vi "HighLvCtrl_Loop.vi"(7 "Processor (-2:auto)":i32=-2, 8 "error in (no error)":errorcluster, 11 "Cluster":T4) -> (0 "error out":errorcluster)   [LabVIEW 2015]
uses:
  Classes/CAlex2/CAlex2.lvclass
  Classes/ForceField/ForceField.lvclass
  <vilib>/Analysis/Matrix/Datatypes/RealMatrix.ctl
  <vilib>/Platform/TimedLoop/XDataNode/timing_clust.ctl
  <vilib>/Platform/TimedLoop/XDataNode/nitl_modes.ctl
  <vilib>/Platform/TimedLoop/XDataNode/wakeup.ctl
  Classes/CAlex2/TypeDef/LowerBodyDim.ctl
  Classes/ForceField/TypeDef/FF_Gains.ctl
  Classes/MotorControl/TypeDef/MotorMode.ctl
  Classes/ForceField/FF_SetGains.vi
  <vilib>/Platform/TimedLoop/XDataNode/XDataNode.xnode
  <vilib>/Platform/TimedLoop/XDataNode/XDNodeRunTimeDep.lvlib
  Classes/SerialChain-Cable/SerialChain-Cable.lvclass
  <vilib>/Analysis/NI_AALBase.lvlib
  <vilib>/Analysis/Matrix/NI_Matrix.lvlib
  <vilib>/GoldZinc Software/auzn custom VIs/CustomVI.lvlib
  <vilib>/Analysis/baseanly.llb/A x Vector.vi
panel:
  in  "history length (100)":i32=50
  in  "Thigh Reference (to Hip)":enum16{"Hip", "Ground"}(ring)=enum."Ground"
  in  "LP":bool
  out "QPSolved":bool
  out "Torque Error":dbl[](array[numeric]) format="%#.4f"
  in  "dt":dbl=0.01 format="%#_13g"
  out "Torque":T1(graph)
  out "Joint Angles (deg)":T2(graph)
  out "Desired Torque":dbl[](array[numeric]) format="%#.4f"
  out "Actual Torque":dbl[](array[numeric]) format="%#.4f"
  in  "LockedJoints":i32[](array[numeric])=[2, 1]
  out "Jacobian for Cables":T3 format="%#.3f"
  in  "TargetF(N)":dbl=15.0 format="%#_13g"
  in  "LP fc":dbl=10.0 format="%0.3f"
  in  "QPmode":enum16{"tight", "loose", "adv"}(ring)=enum."adv"
  in  "F range":cluster{"Fmin":dbl, "Fmax":dbl}[](array[cluster])=[{"Fmin"=15.0, "Fmax"=80.0}, {"Fmin"=10.0, "Fmax"=80.0}, {"Fmin"=10.0, "Fmax"=80.0}, {"Fmin"=10.0, "Fmax"=80.0}]
  # "In Cable Order, Not Motor Order"
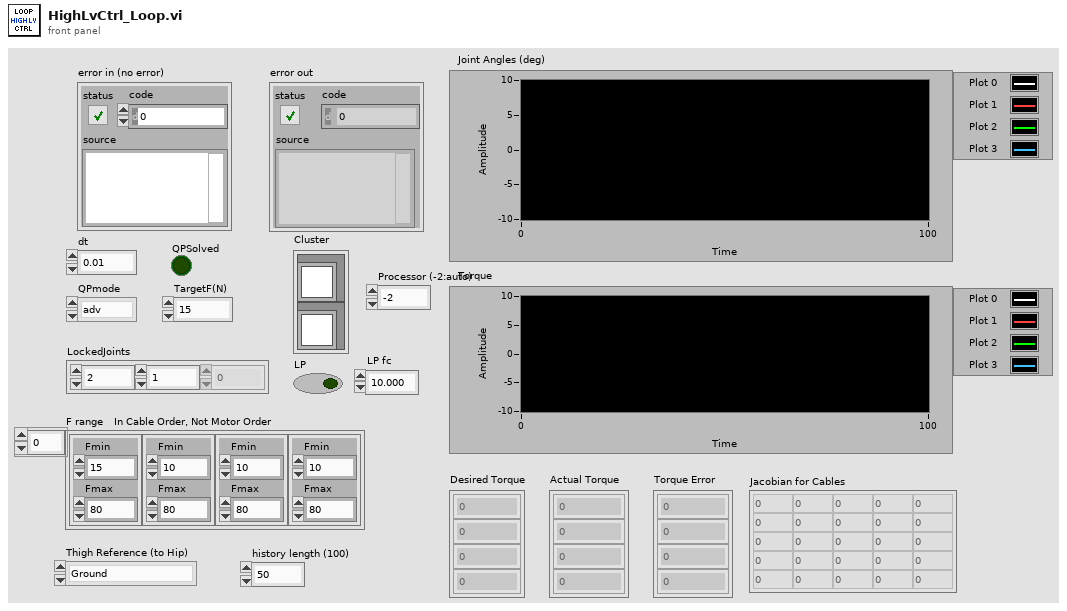
[diagram p1: front panel]
types:
  T1 = cluster{"[0]":dbl, "[1]":dbl, "[2]":dbl, "[3]":dbl, "[4]":dbl, "[5]":dbl, "[6]":dbl, "[7]":dbl, "[8]":dbl}
  T2 = cluster{"Joint Angles (rad)[0]":dbl, "Joint Angles (rad)[1]":dbl, "Joint Angles (rad)[2]":dbl, "Joint Angles (rad)[3]":dbl}
  T3 = typedef "NI_Matrix.lvlib/RealMatrix.ctl" = dbl[][]
  T4 = cluster{"CAlex":refnum<class "CAlex2.lvclass">, "ForceField":refnum<class "ForceField.lvclass">}
  T5 = typedef "XDNodeRunTimeDep.lvlib/timing_clust.ctl" = cluster{"Expected End [f-1]":u64, "Actual End [f-1]":u64, "Finished Late? [f-1]":bool, "Expected End [i-1]":u64, "Actual End [i-1]":u64, "Finished Late? [i-1]":bool, "Expected Start [i]":u64, "Actual Start [i]":u64, "Expected Start [f]":u64, "Actual Start [f]":u64, "Source Name":string, "Structure Name":string, "Period":i64, "Deadline":i64, "Offset":i64, "Start":i64, "Priority":i32, "Timeout":i32, "Mode":T6, "Wakeup Reason":T7, "Error":errorcluster, "Source Type":string, "Secondary Source Type":string, "Global End Time":u64, "Global Start Time":u64, "Frame Duration":u64, "Iteration Duration":u64, "Assigned CPU":i32, "I/O Scan Engine Mode":u32}
  T6 = typedef "XDNodeRunTimeDep.lvlib/nitl_modes.ctl" = enum32{"No Change", "Process missed periods, maintain original phase", "Discard missed periods, maintain original phase", "Process missed periods, ignore original phase", "Discard missed periods, ignore original phase"}
  T7 = typedef "XDNodeRunTimeDep.lvlib/wakeup.ctl" = enum32{"Normal", "Aborted", "Asynchronous wakeup", "Timing source error", "Timed loop error", "Timeout"}
  T8 = typedef "ForceField.lvclass/FF_Gains.ctl" = cluster{"Kn":dbl, "Dn":dbl, "Kt":dbl, "Dt":dbl, "Kd":dbl, "Ns":dbl}
  T9 = typedef "CAlex2.lvclass/LowerBodyDim.ctl" = cluster{"BodyDim":cluster{"ThighLt (m)":dbl, "ShankLt (m)":dbl, "HipWd (m)":dbl}, "BodyWt":cluster{"Thigh (kg)":dbl, "Shank (kg)":dbl}, "Cuff Loc":cluster{"HipCuffWd (m)":dbl, "HipCuffHt (m)":dbl, "HipFwdShift (m)":dbl, "ThighToKnee (m)":dbl, "ThighCuffDist (m)":dbl, "ShankToKnee (m)":dbl}}
  T10 = typedef "SerialChain.lvclass/PointOnBody.ctl" = cluster{"Coord4":dbl[], "ID":i32}
  T11 = cluster{"EndEffPos":T10, "Array of Double":dbl[]}
  T12 = typedef "MotorControl.lvclass/MotorMode.ctl" = enum16{"Idle", "FF", "PID"}
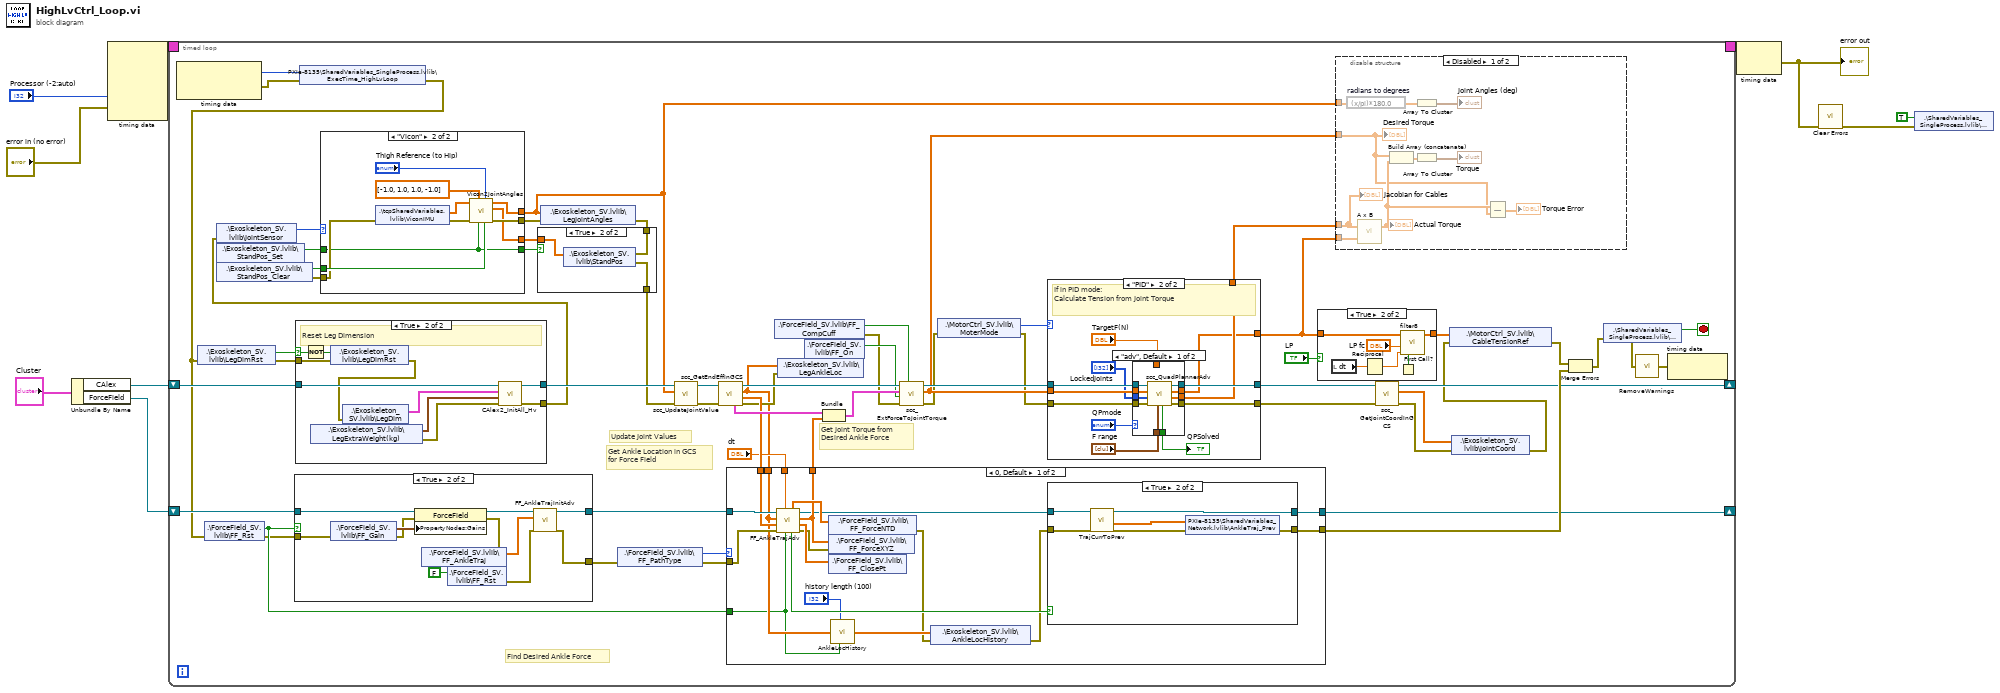
[diagram p0: block diagram]
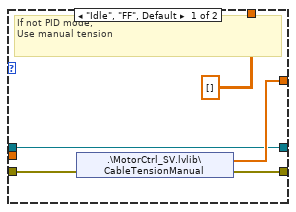
[diagram p4: hidden frame]
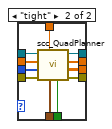
[diagram p5: hidden frame]
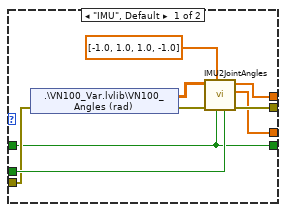
[diagram p6: hidden frame]
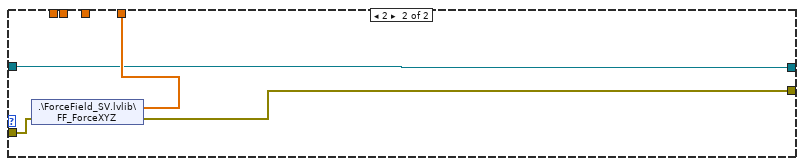
[diagram p11: hidden frame]
diagram:
  n1 = Unbundle By Name("Cluster") -> ("CAlex"=w6:refnum<class "CAlex2.lvclass">, "ForceField"=w5:refnum<class "ForceField.lvclass">)
  n2 = node-c288("Processor (-2:auto)", "error in (no error)") -> (w10:T5)  [unwired: 3 in]
  n3 = timed-loop {
    timing: w10 -> [_]
    timing-out: [_] -> w9
    shift-right: [w15] -> _
    shift-left: w6 -> [w74]
    shift-right: [w36] -> _
    shift-left: w5 -> [w71]
    stop <- w38 stop-if-true
    # "Get Joint Torque from Desired Ankle Force"
    # "Find Desired Ankle Force"
    # "Get Ankle Location in GCS for Force Field"
    # "Update Joint Values"
    n4 = node-c288() -> (w73:i64, w72:errorcluster)  [unwired: 1 in]
    n5 = shared-variable "PXIe-8135\\SharedVariables_SingleProcess.lvlib\\ExecTime_HighLvLoop"(w73, error in=w72) -> (error out=w33:errorcluster)
    n6 = shared-variable ".\\Exoskeleton_SV.lvlib\\LegDimRst"(error in=w33) -> (w52:bool, error out=w66:errorcluster)
    n7 = shared-variable ".\\ForceField_SV.lvlib\\FF_Rst"(error in=w33) -> (w49:bool, error out=w48:errorcluster)
    n8 = case shown="True" w49 {
      tunnel: w71 -> [w154 w166]
      tunnel: [w154 w165] -> w65
      tunnel: w48 -> [w153 w161]
      tunnel: [w153 w155] -> w51
      frame False {
      }
      frame True {
        n9 = shared-variable ".\\ForceField_SV.lvlib\\FF_Gain"(error in=w161) -> (w164:T8, error out=w159:errorcluster)
        n10 = property class="ForceField"(reference=w166, error in=w159, "PropertyNodes:Gains"=w164) -> (reference out=w163:refnum<class "ForceField.lvclass">, error out=w158:errorcluster)
        n11 = shared-variable ".\\ForceField_SV.lvlib\\FF_AnkleTraj"(error in=w158) -> (w162:dbl[][], error out=w157:errorcluster)
        n12 = shared-variable ".\\ForceField_SV.lvlib\\FF_Rst"(FALSE ("FFRst"), error in=w157) -> (error out=w156:errorcluster)
        n13 = call "FF_AnkleTrajInitAdv.vi"("error in (no error)"=w156, "AnkleTraj"=w162, "Force Field Controller in"=w163) -> ("error out"=w155:errorcluster, "Force Field Controller out"=w165:refnum<class "ForceField.lvclass">)  [unwired: 6 in, 1 out]
      }
    }
    n14 = case shown="True" w52 {
      selector: w52 -> [_ w174]
      tunnel: w74 -> [w168 w179]
      tunnel: [w168 w178] -> w67
      tunnel: w66 -> [w167 w177]
      tunnel: [w167 w172] -> w28
      frame False {
      }
      frame True {
        # "Reset Leg Dimension"
        n15 = Not(x=w174) -> (.not. x?=w175:bool)
        n16 = shared-variable ".\\Exoskeleton_SV.lvlib\\LegDimRst"(w175, error in=w177) -> (error out=w171:errorcluster)
        n17 = shared-variable ".\\Exoskeleton_SV.lvlib\\LegDim"(error in=w171) -> (w176:T9, error out=w170:errorcluster)
        n18 = shared-variable ".\\Exoskeleton_SV.lvlib\\LegExtraWeight(kg)"(error in=w170) -> (w173:cluster{"Thigh":dbl, "Shank":dbl}, error out=w169:errorcluster)
        n19 = call-dynamic "CAlex2_InitAll_Hv.vi"("error in (no error)"=w169, "ExtraWeight(kg)"=w173, "LegProperties"=w176, "CAlex2 in"=w179) -> ("error out"=w172:errorcluster, "CAlex2 out"=w178:refnum<class "CAlex2.lvclass">)  [unwired: 6 in]
      }
    }
    n20 = shared-variable ".\\Exoskeleton_SV.lvlib\\JointSensor"(error in=w28) -> (w42:enum16{"IMU", "Vicon"}, error out=w34:errorcluster)
    n21 = shared-variable ".\\Exoskeleton_SV.lvlib\\StandPos_Set"(error in=w34) -> (w53:bool, error out=w40:errorcluster)
    n22 = shared-variable ".\\Exoskeleton_SV.lvlib\\StandPos_Clear"(error in=w40) -> (w54:bool, error out=w41:errorcluster)
    n23 = case shown="\"Vicon\"" w42 {
      tunnel: w54 -> [w129 w141]
      tunnel: w53 -> [w124 w134]
      tunnel: [w128 w139] -> w46
      tunnel: [w127 w142] -> w45
      tunnel: w41 -> [w126 w138]
      tunnel: [w125 w135] -> w24
      tunnel: [w124 w134] -> w23
      frame "IMU", Default {
        n24 = shared-variable ".\\VN100_Var.lvlib\\VN100_Angles (rad)"(error in=w126) -> (w130:dbl[][], error out=w131:errorcluster)
        n25 = call "IMU2JointAngles.vi"("ResetZeroOrient"=w129, "SetZeroOrient"=w124, "JointAngleDir"=dbl[] [-1.0, 1.0, 1.0, -1.0], "error in (no error)"=w131, "IMU in (rad)"=w130) -> ("error out"=w127:errorcluster, "StandPos"=w125:dbl[], "Joint Angles (rad)"=w128:dbl[])  [unwired: 4 in]
      }
      frame "Vicon" {
        n26 = shared-variable ".\\tcpSharedVariables.lvlib\\ViconIMU"(error in=w138) -> (w137:dbl[], error out=w136:errorcluster)
        n27 = call "Vicon2JointAngles.vi"("Reset"=w141, "Thigh Reference (to Hip)"="Thigh Reference (to Hip)", "SetZeroOrient"=w134, "JointAngleDir([-1,1,1,-1])"=dbl[] [-1.0, 1.0, 1.0, -1.0], "error in (no error)"=w136, "ViconIMU in (rad)"=w137) -> ("error out"=w142:errorcluster, "StandPos"=w135:dbl[], "Joint Angles (rad)"=w139:dbl[])  [unwired: 3 in]
      }
    }
    n28 = shared-variable ".\\Exoskeleton_SV.lvlib\\LegJointAngles"(w46, error in=w45) -> (error out=w26:errorcluster)
    n29 = case shown="True" w23 {
      tunnel: w26 -> [w82 w85]
      tunnel: [w82 w84] -> w25
      tunnel: w24 -> [_ w83]
      frame False {
      }
      frame True {
        n30 = shared-variable ".\\Exoskeleton_SV.lvlib\\StandPos"(w83, error in=w85) -> (error out=w84:errorcluster)
      }
    }
    n31 = shared-variable ".\\ForceField_SV.lvlib\\FF_PathType"(error in=w51) -> (w61:i8, error out=w60:errorcluster)
    n32 = call-dynamic "scc_UpdateJointValue.vi"("error in (no error)"=w25, "JointValue (rad|m)"=w46, "C-Alex in"=w67) -> ("error out"=w18:errorcluster, "C-Alex out"=w19:refnum<class "CAlex2.lvclass">)  [unwired: 7 in]
    n33 = call "scc_GetEndEffInGCS.vi"("error in (no error)"=w18, "SerialChain_Cable in"=w19) -> ("error out"=w50:errorcluster, "Vendeff(GCS)"=w62:dbl[], "Pendeff(GCS)"=w11:dbl[], "SerialChain_Cable out"=w69:refnum<class "CAlex2.lvclass">, "EndEffPos"=w70:T10)  [unwired: 5 in]
    n34 = case shown="0, Default" w61 {
      tunnel: w65 -> [w199 w210]
      tunnel: w60 -> [w195 w209]
      tunnel: [w188 w210] -> w36
      tunnel: [w194 w211] -> w63
      tunnel: w11 -> [w184 _]
      tunnel: w62 -> [w191 _]
      tunnel: "dt" -> [w190 _]
      tunnel: w49 -> [w183 _]
      tunnel: [w187 w208] -> w37
      frame 0, Default {
        n35 = call "FF_AnkleTrajAdv.vi"("Init"=w183, "dt"=w190, "error in (no error)"=w195, "AnkleVelocity"=w191, "AnkleInGCS"=w184, "Force Field Controller in"=w199) -> ("error out"=w193:errorcluster, "ClosestPoint"=w197:dbl[], "ForceXYZ"=w194:dbl[], "Force Field Controller out"=w189:refnum<class "ForceField.lvclass">, "UpdateTrajPrev"=w186:bool, "ForceNTD"=w198:dbl[])
        n36 = shared-variable ".\\ForceField_SV.lvlib\\FF_ForceXYZ"(w194, error in=w193) -> (error out=w192:errorcluster)
        n37 = shared-variable ".\\ForceField_SV.lvlib\\FF_ClosePt"(w197, error in=w192) -> (error out=w196:errorcluster)
        n38 = shared-variable ".\\ForceField_SV.lvlib\\FF_ForceNTD"(w198, error in=w196) -> (error out=w182:errorcluster)
        n39 = call "AnkleLocHistory.vi"("history length (100)"="history length (100)", "AnkleLoc"=w184, "initialize"=w183) -> ("AnkleLoc"=w185:dbl[][])  [unwired: 2 in]
        n40 = shared-variable ".\\Exoskeleton_SV.lvlib\\AnkleLocHistory"(w185, error in=w182) -> (error out=w181:errorcluster)
        n41 = case shown="True" w186 {
          tunnel: w189 -> [w201 w206]
          tunnel: [w201 w207] -> w188
          tunnel: w181 -> [w200 w204]
          tunnel: [w200 w202] -> w187
          frame False {
          }
          frame True {
            n42 = call "TrajCurrToPrev.vi"("error in (no error)"=w204, "ForceField"=w206) -> ("error out"=w203:errorcluster, "AnkleTraj_array"=w205:dbl[][], "ForceField 2"=w207:refnum<class "ForceField.lvclass">)  [unwired: 6 in, 1 out]
            n43 = shared-variable "PXIe-8135\\SharedVariables_Network.lvlib\\AnkleTraj_Prev"(w205, error in=w203) -> (error out=w202:errorcluster)
          }
        }
      }
      frame 2 {
        n44 = shared-variable ".\\ForceField_SV.lvlib\\FF_ForceXYZ"(error in=w209) -> (w211:dbl[], error out=w208:errorcluster)
      }
    }
    n45 = shared-variable ".\\Exoskeleton_SV.lvlib\\LegAnkleLoc"(w11, error in=w50) -> (error out=w58:errorcluster)
    n46 = shared-variable ".\\ForceField_SV.lvlib\\FF_On"(error in=w58) -> (w57:bool, error out=w59:errorcluster)
    n47 = shared-variable ".\\ForceField_SV.lvlib\\FF_CompCuff"(error in=w59) -> (w35:bool, error out=w56:errorcluster)
    n48 = Bundle("EndEffPos"=w70, "Array of Double"=w63) -> (w64:T11)  [unwired: 1 in]
    n49 = call "scc_ExtForceToJointTorque.vi"("CuffWtComp?(F)"=w35, "error in (no error)"=w56, "ExternalForce(T)"=w57, "External Force (In GCS)"=w64, "SerialChain_Cable in"=w69) -> ("error out"=w29:errorcluster, "DesiredTorque(Nm)"=w44:dbl[], "SerialChain_Cable out"=w68:refnum<class "CAlex2.lvclass">)  [unwired: 4 in]
    n50 = shared-variable ".\\MotorCtrl_SV.lvlib\\MoterMode"(error in=w29) -> (w31:T12, error out=w30:errorcluster)
    n51 = case shown="\"PID\"" w31 {
      tunnel: [w89 w102] -> w17
      tunnel: w30 -> [w88 w101]
      tunnel: w68 -> [w89 w100]
      tunnel: [T3 [] ("Jacobian for Cables") w96] -> w47
      tunnel: w44 -> [_ w95]
      tunnel: [w90 w94] -> w32
      tunnel: [w87 w93] -> w16
      frame "Idle", "FF", Default {
        # "If not PID mode,\nUse manual tension"
        n52 = shared-variable ".\\MotorCtrl_SV.lvlib\\CableTensionManual"(error in=w88) -> (w90:dbl[], error out=w87:errorcluster)
      }
      frame "PID" {
        # "If in PID mode:\nCalculate Tension from Joint Torque"
        n53 = case shown="\"adv\", Default" "QPmode" {
          tunnel: w101 -> [w105 w123]
          tunnel: w100 -> [w111 w122]
          tunnel: w95 -> [w110 w115]
          tunnel: [w112 w121] -> w102
          tunnel: "F range" -> [w107 w120]
          tunnel: [w106 w119] -> w99
          tunnel: [w109 w118] -> w94
          tunnel: [w108 w117] -> w93
          tunnel: "TargetF(N)" -> [_ w116]
          tunnel: "LockedJoints" -> [w104 w114]
          tunnel: [w103 w113] -> w96
          frame "adv", Default {
            n54 = call "scc_QuadPlannerAdv.vi"("F range (of each cable)"=w107, "error in (no error)"=w105, "LockedJoint(StartFrom0)"=w104, "DesireTorque(Nm)"=w110, "SerialChain_Cable in"=w111) -> ("error out"=w108:errorcluster, "Jacobian for Cables"=w103:T3, "Planned Tension"=w109:dbl[], "SerialChain_Cable out"=w112:refnum<class "CAlex2.lvclass">, "Solved"=w106:bool)  [unwired: 2 in]
          }
          frame "tight" {
            n55 = call "scc_QuadPlanner.vi"("F range"=w120, "TargetF(N)"=w116, "error in (no error)"=w123, "LockedJoint(StartFrom0)"=w114, "DesireTorque(Nm)"=w115, "SerialChain_Cable in"=w122) -> ("error out"=w117:errorcluster, "Jacobian for Cables"=w113:T3, "Planned Tension"=w118:dbl[], "SerialChain_Cable out"=w121:refnum<class "CAlex2.lvclass">, "Solved"=w119:bool)  [unwired: 1 in]
          }
        }
        "QPSolved" <- w99
      }
    }
    n56 = case shown="True" "LP" {
      tunnel: w32 -> [w75 w78]
      tunnel: [w75 w77] -> w27
      frame False {
      }
      frame True {
        n57 = local read "dt"() -> (w80:dbl)
        n58 = Reciprocal(x=w80) -> (1/x=w79:dbl)
        n59 = First Call?() -> (First Call?: T/F=w76:bool)
        n60 = call "filter8.vi"("initialize"=w76, "sampling freq: fs"=w79, "low cutoff freq: fl"="LP fc", "Array"=w78) -> ("appended array"=w77:dbl[])  [unwired: 7 in]
      }
    }
    n61 = disable-structure shown="Disabled" {
      disable-tunnel: w47 -> [w152 _]
      disable-tunnel: w32 -> [w151 _]
      disable-tunnel: w46 -> [w150 _]
      disable-tunnel: w44 -> [w144 _]
      frame Disabled {
        n62 = expression code="(x/pi)*180.0" "radians to degrees"(w150) -> (w147:dbl[])
        n63 = call-poly <vilib>:"A x B.vi"("Vector"=w151, "A"=w152) -> ("A x Vector"=w145:dbl[])  [unwired: 1 out]
        "Actual Torque" <- w145
        n64 = Build Array (concatenate)(w144, w145) -> (w148:dbl[])
        n65 = Array To Cluster(array=w147) -> (cluster=→"Joint Angles (deg)":T2)
        n66 = Array To Cluster(array=w148) -> (cluster=→"Torque":T1)
        n67 = Subtract(x=w145, y=w144) -> (x-y=→"Torque Error":dbl[])
        "Jacobian for Cables" <- w152
        "Desired Torque" <- w144
      }
      frame Enabled {
      }
    }
    n68 = call "scc_GetJointCoordInGCS.vi"("error in (no error)"=w16, "SerialChain_Cable in"=w17) -> ("error out"=w13:errorcluster, "Joint Coord in GCS"=w14:dbl[][], "SerialChain_Cable out"=w15:refnum<class "CAlex2.lvclass">)  [unwired: 5 in, 2 out]
    n69 = shared-variable ".\\Exoskeleton_SV.lvlib\\JointCoord"(w14, error in=w13) -> (error out=w12:errorcluster)
    n70 = shared-variable ".\\MotorCtrl_SV.lvlib\\CableTensionRef"(w27, error in=w12) -> (error out=w43:errorcluster)
    n71 = Merge Errors(w43, w37) -> (w39:errorcluster)
    n72 = shared-variable ".\\SharedVariables_SingleProcess.lvlib\\GlobalStop"(error in=w39) -> (w38:bool, error out=w22:errorcluster)
    n73 = call <vilib>:"RemoveWarnings.vi"("error in (no error)"=w22) -> ("error out"=w21:errorcluster)
    n74 = node-c288(w21) -> ()  [unwired: 1 out]
  }
  n75 = node-c288(w9) -> (w3:errorcluster)
  "error out" <- w3
  n76 = call <vilib>:"Clear Errors.vi"("error in (no error)"=w3) -> ("error out"=w2:errorcluster)  [unwired: 5 in, 1 out]
  n77 = shared-variable ".\\SharedVariables_SingleProcess.lvlib\\GlobalStop"(TRUE ("GlobalStop"), error in=w2) -> ()  [unwired: 1 out]
